vi "Stage 1.1 myDAQ - getting it working.vi"() -> ()   [LabVIEW 2020]
uses:
  <vilib>/DAQmx/read.llb/DAQmx Read (Analog 1D DBL 1Chan NSamp).vi
  <vilib>/DAQmx/create/channels.llb/DAQmx Create Channel (AI-Voltage-Basic).vi
  <vilib>/DAQmx/configure/timing.llb/DAQmx Timing (Sample Clock).vi
  <vilib>/DAQmx/miscellaneous.llb/DAQmx Fill In Error Info.vi
panel:
  out "error out":errorcluster
  out "Waveform Chart":dbl[](graph)
  in  "Stop":bool
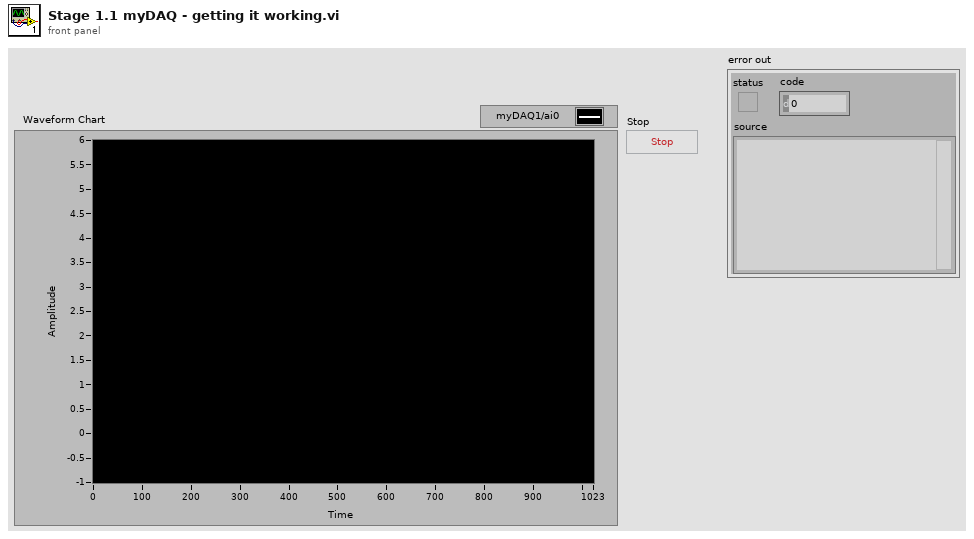
[diagram p1: front panel]
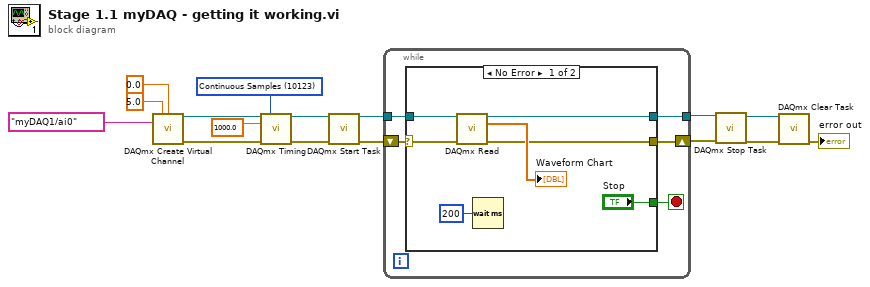
[diagram p0: block diagram]
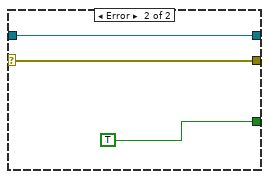
[diagram p2: hidden frame]
diagram:
  w13 = 10123 items=["Finite Samples"=10178, "Continuous Samples"=10123, "Hardware Timed Single Point"=12522] ("sample mode")
  n1 = call-poly <vilib>:"DAQmx Create Virtual Channel.vi"("maximum value"=5.0, "minimum value"=0.0, "physical channels"=tag "myDAQ1/ai0") -> ("task out"=w16:refnum<k21>, "error out"=w15:errorcluster)  [unwired: 11 in]
  n2 = call-poly <vilib>:"DAQmx Timing.vi"("task/channels in"=w16, "sample mode"=w13, "rate"=1000.0, "error in"=w15) -> ("task out"=w7:refnum<k21>, "error out"=w10:errorcluster)  [unwired: 10 in]
  n3 = call <vilib>:"DAQmx Start Task.vi"("task/channels in"=w7, "error in"=w10) -> ("task out"=w8:refnum<k21>, "error out"=w9:errorcluster)  [unwired: 12 in]
  n4 = while {
    tunnel: w8 -> [w21]
    tunnel: [w19] -> w4
    shift-right: [w18] -> w3
    shift-left: w9 -> [w20]
    stop <- w17 stop-if-true
    n5 = case shown="No Error" w20 {
      selector: w20 -> [w27 w30]
      tunnel: w21 -> [w28 w29]
      tunnel: [w24 w29] -> w19
      tunnel: [w23 w30] -> w18
      tunnel: ["Stop" TRUE ("Stop")] -> w17
      frame No Error {
        n6 = call-poly <vilib>:"DAQmx Read.vi"("task/channels in"=w28, "error in"=w27) -> ("task out"=w24:refnum<k21>, "data"=→"Waveform Chart":dbl[], "error out"=w23:errorcluster)  [unwired: 11 in]
        n7 = Wait (ms)(milliseconds to wait=u32 200) -> ()  [unwired: 1 out]
      }
      frame Error {
      }
    }
  }
  n8 = call <vilib>:"DAQmx Stop Task.vi"("task/channels in"=w4, "error in"=w3) -> ("task out"=w6:refnum<k21>, "error out"=w5:errorcluster)  [unwired: 12 in]
  n9 = call <vilib>:"DAQmx Clear Task.vi"("task in"=w6, "error in"=w5) -> ("error out"=→"error out":errorcluster)  [unwired: 13 in]
